vi "Spectrometer_R&S_2017.03.17.vi"(6 "ESR_stack_ref":refnum<vi>, 8 "current_run_ref":refnum<vi>, 9 "generator_enable":bool, 10 "sweep_parameters":T1={"Repetitions"=1, "Power dBm"=5.999999061226845, "Freq Start [Hz]"=2800000000.0, "Freq Stop [Hz]"=3000000000.0, "Step size [Hz]"=2500000.0, "Dwell Time [ms]"=0.09999999974525053} {"Dwell Time [ms]" format="%.3f"; "Step size [Hz]" format="%.2p"; "Freq Stop [Hz]" format="%.2p"; "Freq Start [Hz]" format="%.2p"; "Power dBm" format="%.2f"; "Repetitions" min=1 max=1000 step=1}, 11 "position_xyz":T2 {"Position Z" min=0.0 max=10.0 step=0.001 format="%.3f"; "Position Y" min=-10.0 max=10.0 step=0.1 format="%.3f"; "Position X" min=-10.0 max=10.0 step=0.1 format="%.3f"}) -> ()   [LabVIEW 2014]
uses:
  <vilib>/DAQmx/write.llb/DAQmx Write (Digital Bool 1Line 1Point).vi
  <vilib>/Analysis/baseanly.llb/Vector x A.vi
  GLOBAL_VAR.vi
  <vilib>/DAQmx/miscellaneous.llb/DAQmx Fill In Error Info.vi
  <vilib>/Analysis/Matrix/Numeric/Conversions/Array To Matrix - RA2.vi
  <vilib>/DAQmx/create/channels.llb/DAQmx Create Channel (CO-Pulse Generation-Ticks).vi
  <vilib>/DAQmx/create/channels.llb/DAQmx Create Channel (DO-Digital Output).vi
  <vilib>/DAQmx/create/channels.llb/DAQmx Create Channel (AO-Voltage-Basic).vi
  <vilib>/DAQmx/configure/trigger.llb/DAQmx Start Trigger (Digital Edge).vi
  <resource>/objmgr/daqmx.rc
  <vilib>/Analysis/NI_AALBase.lvlib
  <vilib>/Analysis/Matrix/NI_Matrix.lvlib
  <instrlib>/Rohde&Schwarz RF Signal Generator/Rohde&Schwarz RF Signal Generator.lvlib
  <vilib>/DAQmx/write.llb/DAQmx Write (Analog 1D DBL NChan 1Samp).vi
panel:
  out "File name":string
  in  "Save":bool
  in  "Stop":bool
  out "Run":i32=100
  out "Remain":i32
  out "Intensity Graph":ext[][](graph)
  out "Histogram":cluster{ext[], ext[]}[](graph)=[{[2700000000.0, 2702500000.0, 2705000000.0, 2707500000.0, 2710000000.0, 2712500000.0, 2715000000.0, 2717500000.0, 2720000000.0, 2722500000.0, 2725000000.0, 2727500000.0, 2730000000.0, 2732500000.0, 2735000000.0, 2737500000.0, 2740000000.0, 2742500000.0, 2745000000.0, 2747500000.0, 2750000000.0, 2752500000.0, 2755000000.0, 2757500000.0, 2760000000.0, 2762500000.0, 2765000000.0, 2767500000.0, 2770000000.0, 2772500000.0, 2775000000.0, 2777500000.0, 2780000000.0, 2782500000.0, 2785000000.0, 2787500000.0, 2790000000.0, 2792500000.0, 2795000000.0, 2797500000.0, 2800000000.0, 2802500000.0, 2805000000.0, 2807500000.0, 2810000000.0, 2812500000.0, 2815000000.0, 2817500000.0, 2820000000.0, 2822500000.0, 2825000000.0, 2827500000.0, 2830000000.0, 2832500000.0, 2835000000.0, 2837500000.0, 2840000000.0, 2842500000.0, 2845000000.0, 2847500000.0, 2850000000.0, 2852500000.0, 2855000000.0, 2857500000.0, 2860000000.0, 2862500000.0, 2865000000.0, 2867500000.0, 2870000000.0, 2872500000.0, 2875000000.0, 2877500000.0, 2880000000.0, 2882500000.0, 2885000000.0, 2887500000.0, 2890000000.0, 2892500000.0, 2895000000.0, 2897500000.0, 2900000000.0, 2902500000.0, 2905000000.0, 2907500000.0, 2910000000.0, 2912500000.0, 2915000000.0, 2917500000.0, 2920000000.0, 2922500000.0, 2925000000.0, 2927500000.0, 2930000000.0, 2932500000.0, 2935000000.0, 2937500000.0, 2940000000.0, 2942500000.0, 2945000000.0, 2947500000.0, 2950000000.0, 2952500000.0, 2955000000.0, 2957500000.0, 2960000000.0, 2962500000.0, 2965000000.0, 2967500000.0, 2970000000.0, 2972500000.0, 2975000000.0, 2977500000.0, 2980000000.0, 2982500000.0, 2985000000.0, 2987500000.0, 2990000000.0, 2992500000.0, 2995000000.0, 2997500000.0, 3000000000.0], [26841.121559672197128, 27464.174520667373477, 27576.32405364650522, 29408.099758972323686, 27638.629349746022854, 27576.32405364650522, 27638.629349746022854, 27651.09040896592638, 28398.753962160138, 28311.526547620813311, 28236.76019230139215, 27912.772652583900449, 27850.467356484382814, 27875.389474924189868, 28174.454896201874515, 28697.819383437822648, 28685.35832421791912, 28535.825613579076798, 28809.968916416954391, 29046.729041595121403, 28647.975146558208541, 28523.36455435917327, 28062.305363222742772, 28174.454896201874515, 28473.520317479559163, 27738.31782350525107, 28423.676080599945054, 29133.956456134446093, 28859.8131532965685, 27638.629349746022854, 29133.956456134446093, 27763.239941945058124, 27352.024987688241733, 27439.252402227566423, 28822.429975636857918, 27526.479816766891112, 28548.286672798980325, 27838.006297264479286, 28847.352094076664972, 28884.735271736375553, 29271.02810755338489, 28884.735271736375553, 27289.7196915887241, 28971.962686275700243, 28336.448666060620365, 28548.286672798980325, 27975.077948683418082, 27763.239941945058124, 29470.405055071841321, 28822.429975636857918, 28087.227481662549826, 28286.604429181006259, 27352.024987688241733, 27401.869224567855841, 28398.753962160138, 29308.411285213095471, 28485.98137669946269, 28585.669850458690906, 28710.280442657726175, 28236.76019230139215, 28311.526547620813311, 27576.32405364650522, 27302.180750808627625, 28299.065488400909786, 26878.504737331907709, 28809.968916416954391, 29420.560818192227213, 28859.8131532965685, 27750.778882725154597, 28535.825613579076798, 28398.753962160138, 28261.682310741199204, 28947.040567835893189, 28361.370784500427419, 28785.046797977147337, 28610.59196889849796, 27476.635579887277004, 28062.305363222742772, 28311.526547620813311, 28809.968916416954391, 28647.975146558208541, 28112.14960010235688, 28822.429975636857918, 27738.31782350525107, 28199.377014641681569, 28510.903495139269744, 27451.71346144746995, 28074.766422442646299, 27725.856764285347543, 28635.514087338305014, 28834.891034856761445, 27376.947106128048787, 29096.573278474735512, 28274.143369961102731, 29034.267982375217876, 28560.747732018883852, 27277.258632368820573, 28884.735271736375553, 28049.844304002839245, 27975.077948683418082, 26965.732151871232396, 28809.968916416954391, 28000.000067123225136, 27127.725921729978248, 28037.383244782935718, 28000.000067123225136, 27277.258632368820573, 27800.623119604768705, 28087.227481662549826, 27501.557698327084058, 26778.816263572679492, 26429.906605415380737, 27526.479816766891112, 26442.367664635284264, 26479.750842294994845, 27775.701001164961651, 27040.498507190653559, 26429.906605415380737, 27750.778882725154597, 27464.174520667373477, 27925.233711803803976]}, {[2700000000.0, 2702500000.0, 2705000000.0, 2707500000.0, 2710000000.0, 2712500000.0, 2715000000.0, 2717500000.0, 2720000000.0, 2722500000.0, 2725000000.0, 2727500000.0, 2730000000.0, 2732500000.0, 2735000000.0, 2737500000.0, 2740000000.0, 2742500000.0, 2745000000.0, 2747500000.0, 2750000000.0, 2752500000.0, 2755000000.0, 2757500000.0, 2760000000.0, 2762500000.0, 2765000000.0, 2767500000.0, 2770000000.0, 2772500000.0, 2775000000.0, 2777500000.0, 2780000000.0, 2782500000.0, 2785000000.0, 2787500000.0, 2790000000.0, 2792500000.0, 2795000000.0, 2797500000.0, 2800000000.0, 2802500000.0, 2805000000.0, 2807500000.0, 2810000000.0, 2812500000.0, 2815000000.0, 2817500000.0, 2820000000.0, 2822500000.0, 2825000000.0, 2827500000.0, 2830000000.0, 2832500000.0, 2835000000.0, 2837500000.0, 2840000000.0, 2842500000.0, 2845000000.0, 2847500000.0, 2850000000.0, 2852500000.0, 2855000000.0, 2857500000.0, 2860000000.0, 2862500000.0, 2865000000.0, 2867500000.0, 2870000000.0, 2872500000.0, 2875000000.0, 2877500000.0, 2880000000.0, 2882500000.0, 2885000000.0, 2887500000.0, 2890000000.0, 2892500000.0, 2895000000.0, 2897500000.0, 2900000000.0, 2902500000.0, 2905000000.0, 2907500000.0, 2910000000.0, 2912500000.0, 2915000000.0, 2917500000.0, 2920000000.0, 2922500000.0, 2925000000.0, 2927500000.0, 2930000000.0, 2932500000.0, 2935000000.0, 2937500000.0, 2940000000.0, 2942500000.0, 2945000000.0, 2947500000.0, 2950000000.0, 2952500000.0, 2955000000.0, 2957500000.0, 2960000000.0, 2962500000.0, 2965000000.0, 2967500000.0, 2970000000.0, 2972500000.0, 2975000000.0, 2977500000.0, 2980000000.0, 2982500000.0, 2985000000.0, 2987500000.0, 2990000000.0, 2992500000.0, 2995000000.0, 2997500000.0, 3000000000.0], [27662.305362263847, 27614.704116043806, 27558.75396014644, 27479.62623410005, 27635.264863756656, 27635.514084941045, 27523.73838373851, 27614.704116043802, 27583.17763621744, 27571.58885114293, 27593.520315369973, 27605.109100444486, 27505.545237277456, 27540.685424277577, 27573.831841802512, 27521.74461426332, 27747.788228512374, 27553.395704681883, 27408.099754177805, 27507.040564383846, 27553.769536458476, 27450.09352374888, 27547.16517507192, 27590.529661157172, 27485.98137430221, 27331.838071751987, 27460.06237112481, 27420.436202805507, 27402.99071989765, 27434.64181031619, 27576.697885423117, 27476.38635870286, 27470.654271461714, 27460.311592309215, 27451.962682631867, 27448.722807234688, 27469.781997316335, 27462.056140599987, 27364.23682572375, 27414.081062603364, 27456.573274543232, 27499.688539444087, 27488.598196738385, 27439.252402227583, 27451.215019078678, 27574.45489476352, 27513.894146954794, 27562.741499096825, 27559.377013107456, 27384.42374165998, 27576.074832462113, 27480.747729429848, 27504.423741947663, 27448.099754273695, 27508.90972326683, 27439.50162341197, 27397.383243248685, 27424.54835234809, 27331.21501879102, 27477.258632848276, 27459.68853934821, 27434.267978539607, 27381.05925567063, 27417.07171681613, 27347.912838145676, 27456.82249572762, 27392.398819560723, 27427.539006560855, 27402.86610930546, 27384.79757343659, 27482.86610949723, 27504.049910171063, 27508.037449121424, 27430.778881958024, 27495.202558124915, 27442.367667032533, 27426.16829004667, 27367.60131171313, 27402.616888121054, 27600.00006616432, 27539.68853953999, 27533.58262052224, 27462.305361784383, 27564.361436795392, 27572.087293511737, 27503.55146780227, 27476.137137518494, 27474.766421004293, 27580.560813781274, 27579.813150228085, 27592.024988263576, 27505.296016093063, 27570.84118758975, 27614.953337228195, 27611.215019462234, 27484.236826011424, 27503.925299578863, 27544.54835263575, 27602.616888600503, 27550.903492837893, 27593.769536554377, 27516.63557998317, 27611.962683015438, 27551.028103430108, 27655.701000877292, 27659.688539827646, 27578.5670443061, 27729.59508205134, 27610.093524132444, 27489.968913252564, 27615.202558412602, 27486.479816671, 27421.059255766515, 27418.56704392252, 27449.221249603488, 27600.996950901917, 27543.92529967475, 27425.17140530909, 27466.04367955036, 27523.987604922913, 27501.183866550484]}]
  in  "start":bool
  in  "stop":bool
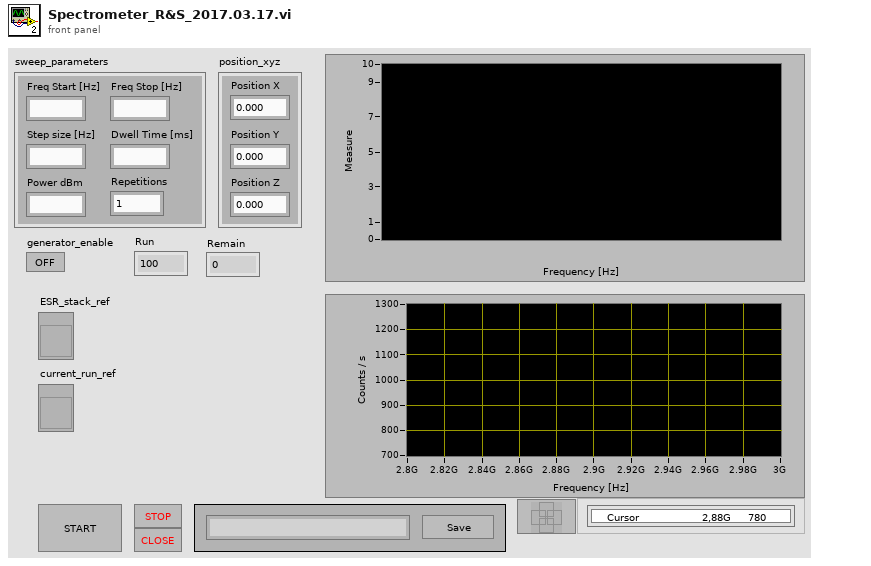
[diagram p1: front panel]
types:
  T1 = cluster{"Repetitions":i32, "Power dBm":ext, "Freq Start [Hz]":ext, "Freq Stop [Hz]":ext, "Step size [Hz]":ext, "Dwell Time [ms]":ext}
  T2 = cluster{"Position X":dbl, "Position Y":dbl, "Position Z":dbl}
  T3 = enum16{"stand-by", "init", "config", "acquisition", "processing", "close", "Set Variables"}
  T4 = typedef "NI_Matrix.lvlib/RealMatrix.ctl" = dbl[][]
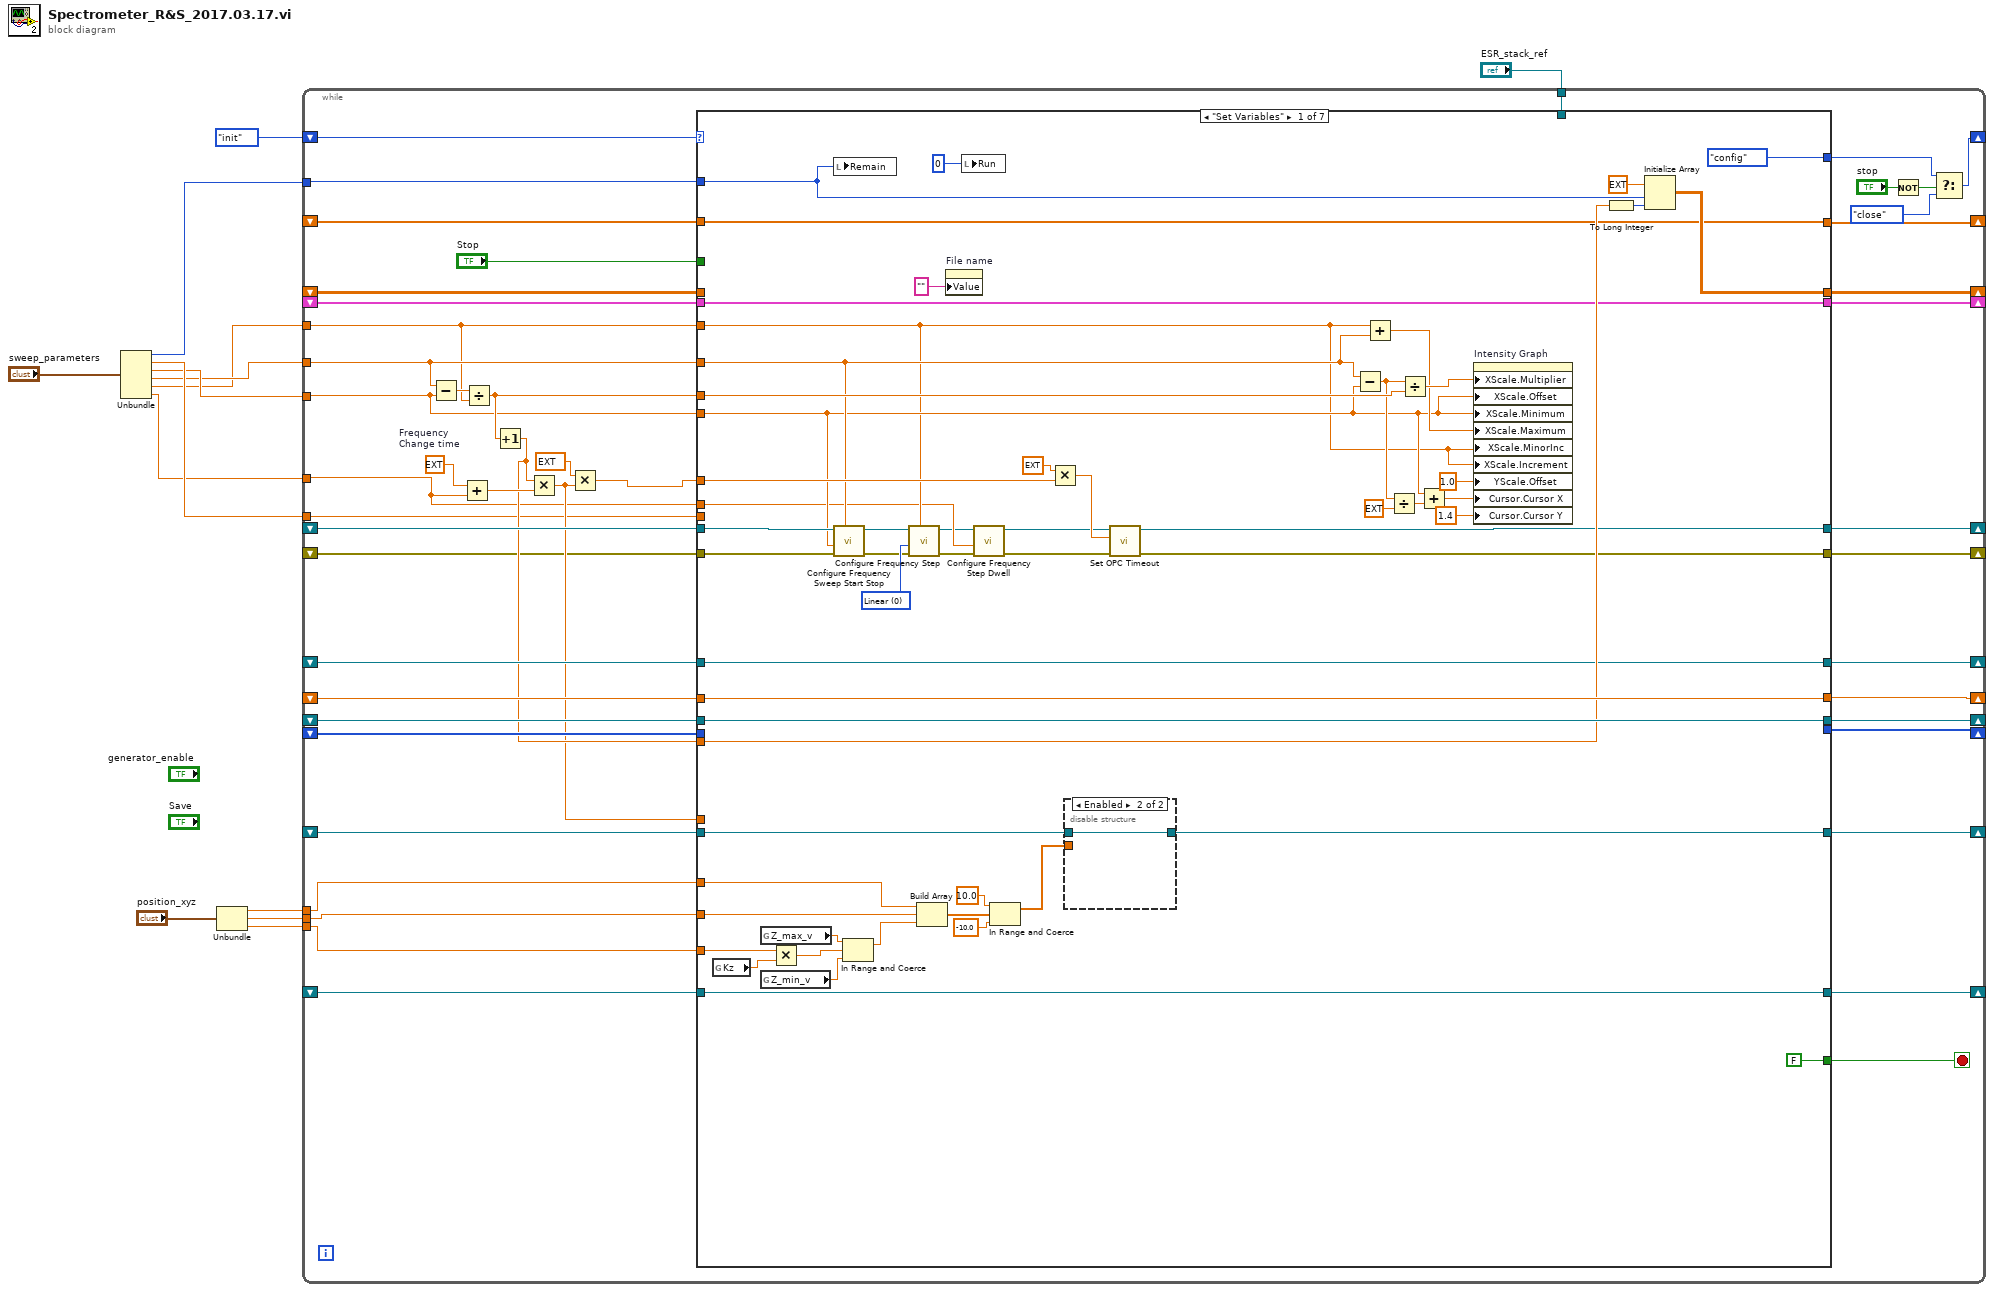
[diagram p0: block diagram]
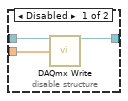
[diagram p2: hidden frame]
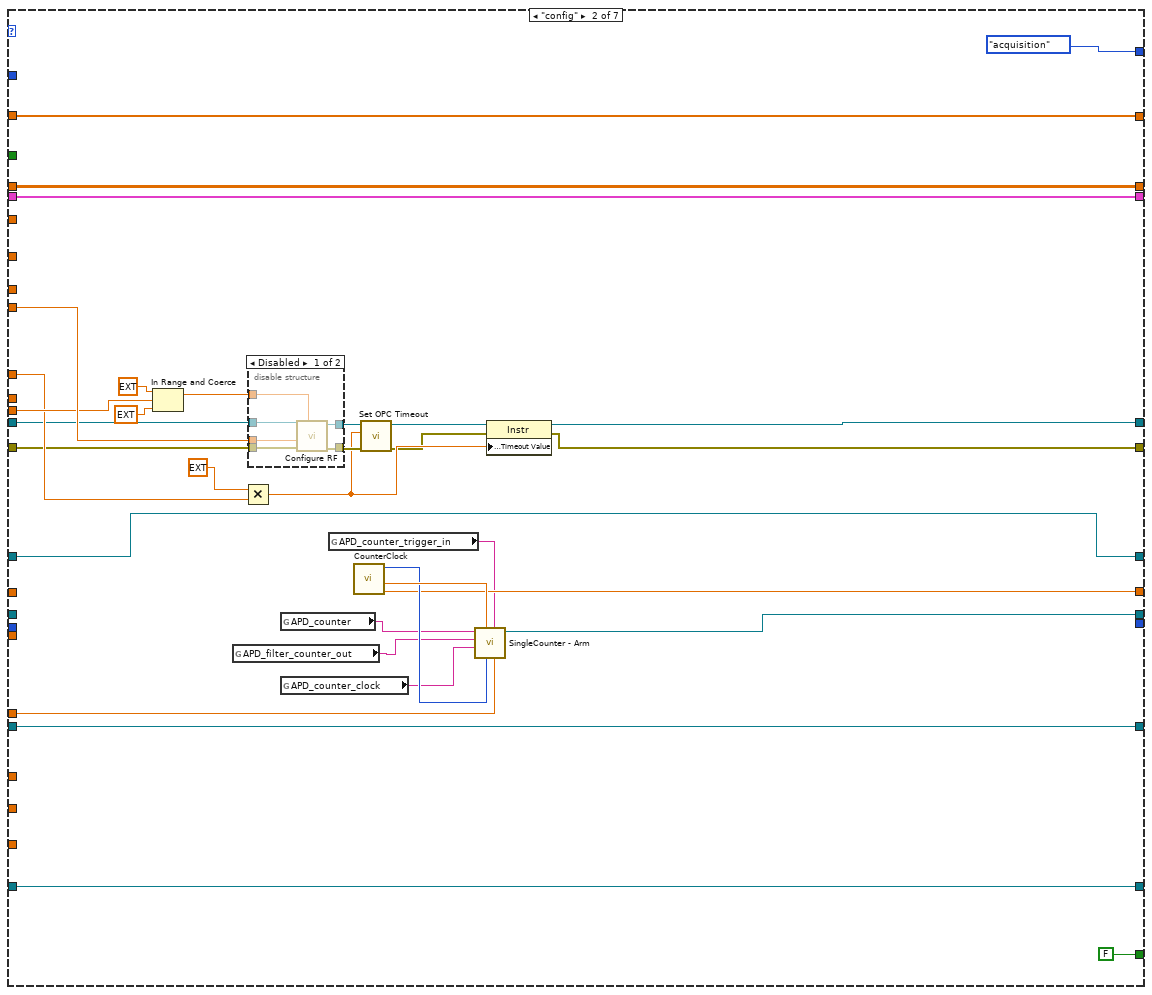
[diagram p3: hidden frame]
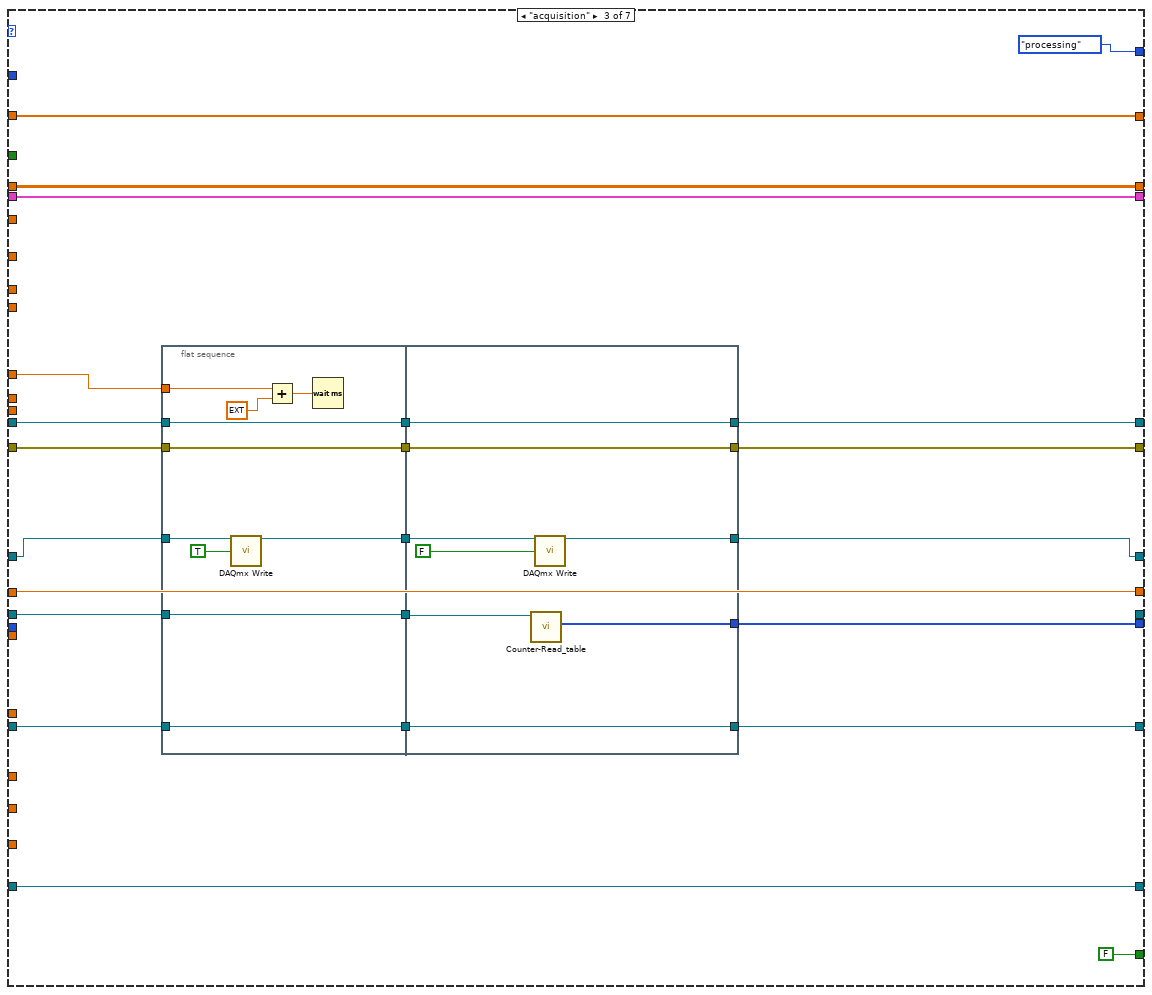
[diagram p5: hidden frame]
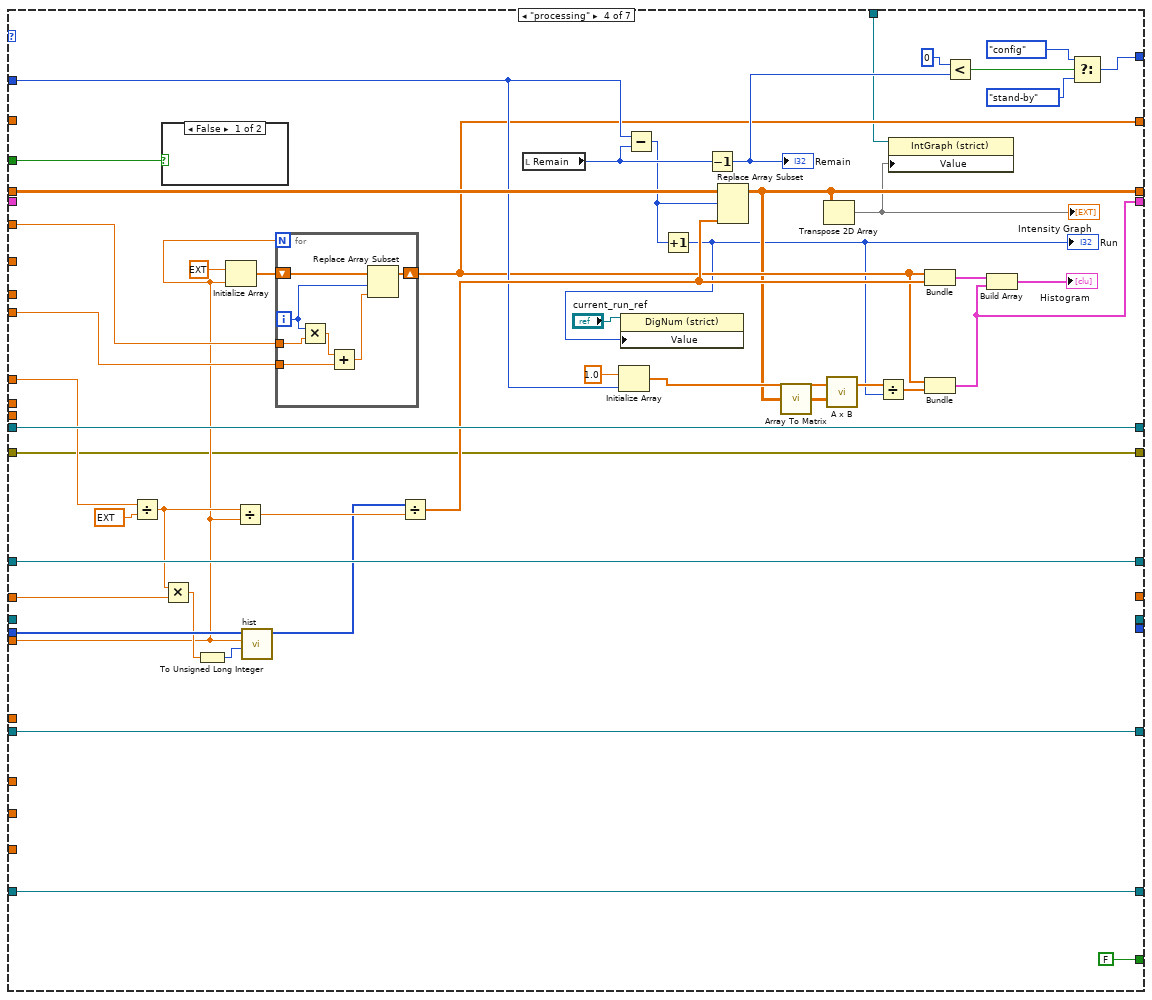
[diagram p6: hidden frame]
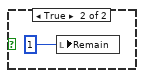
[diagram p7: hidden frame]
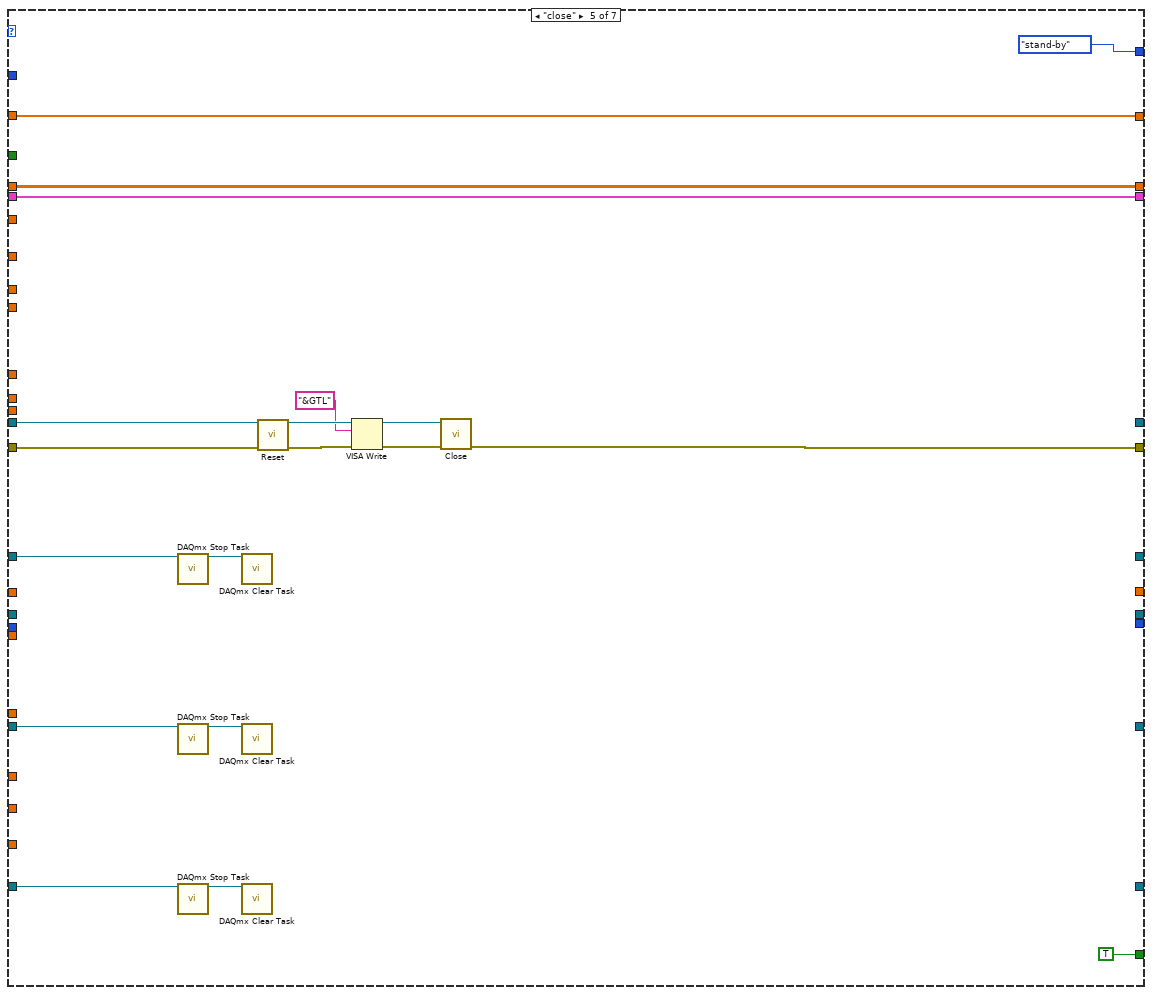
[diagram p8: hidden frame]
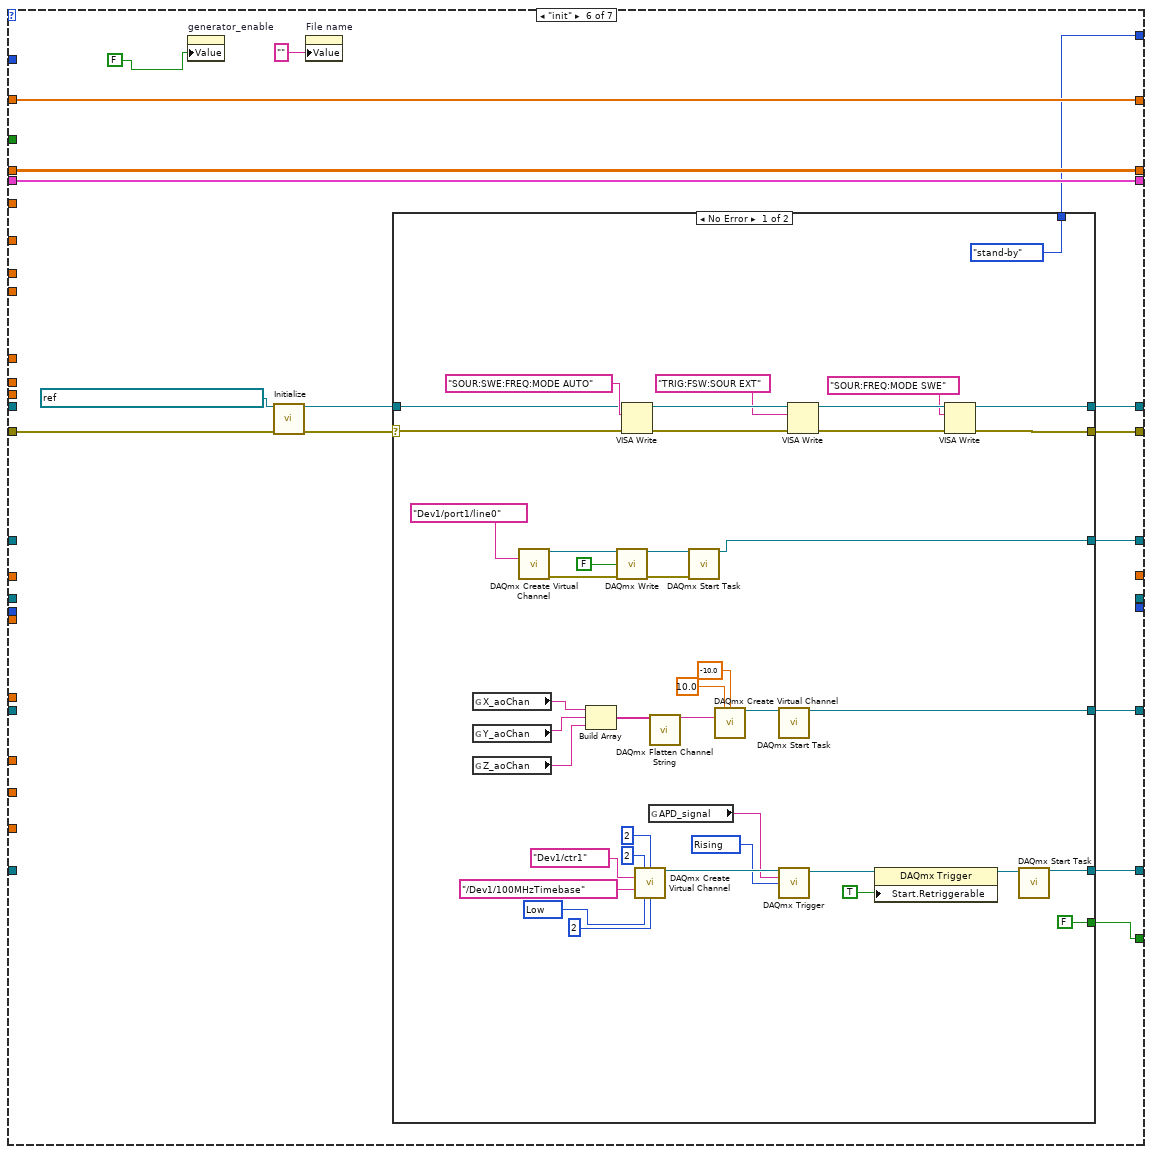
[diagram p9: hidden frame]
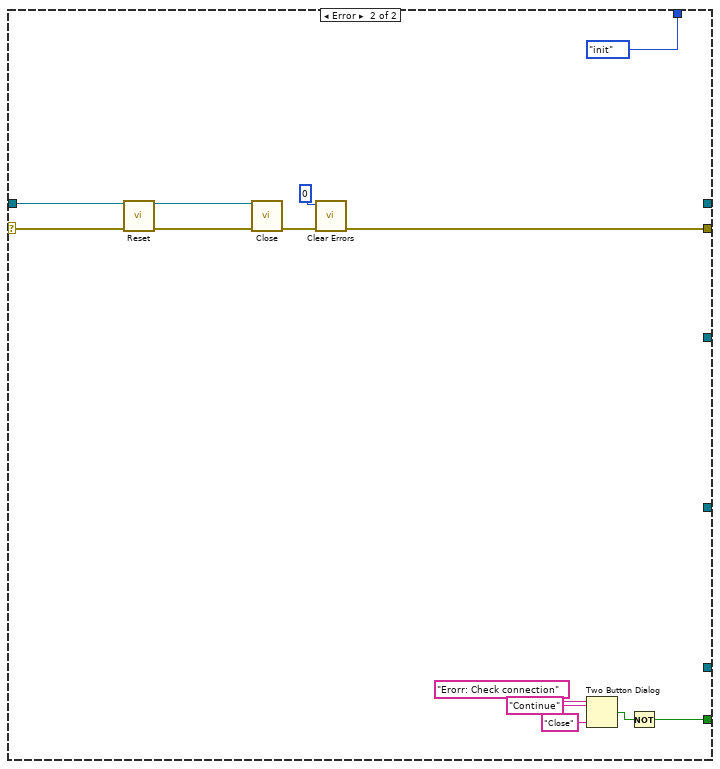
[diagram p10: hidden frame]
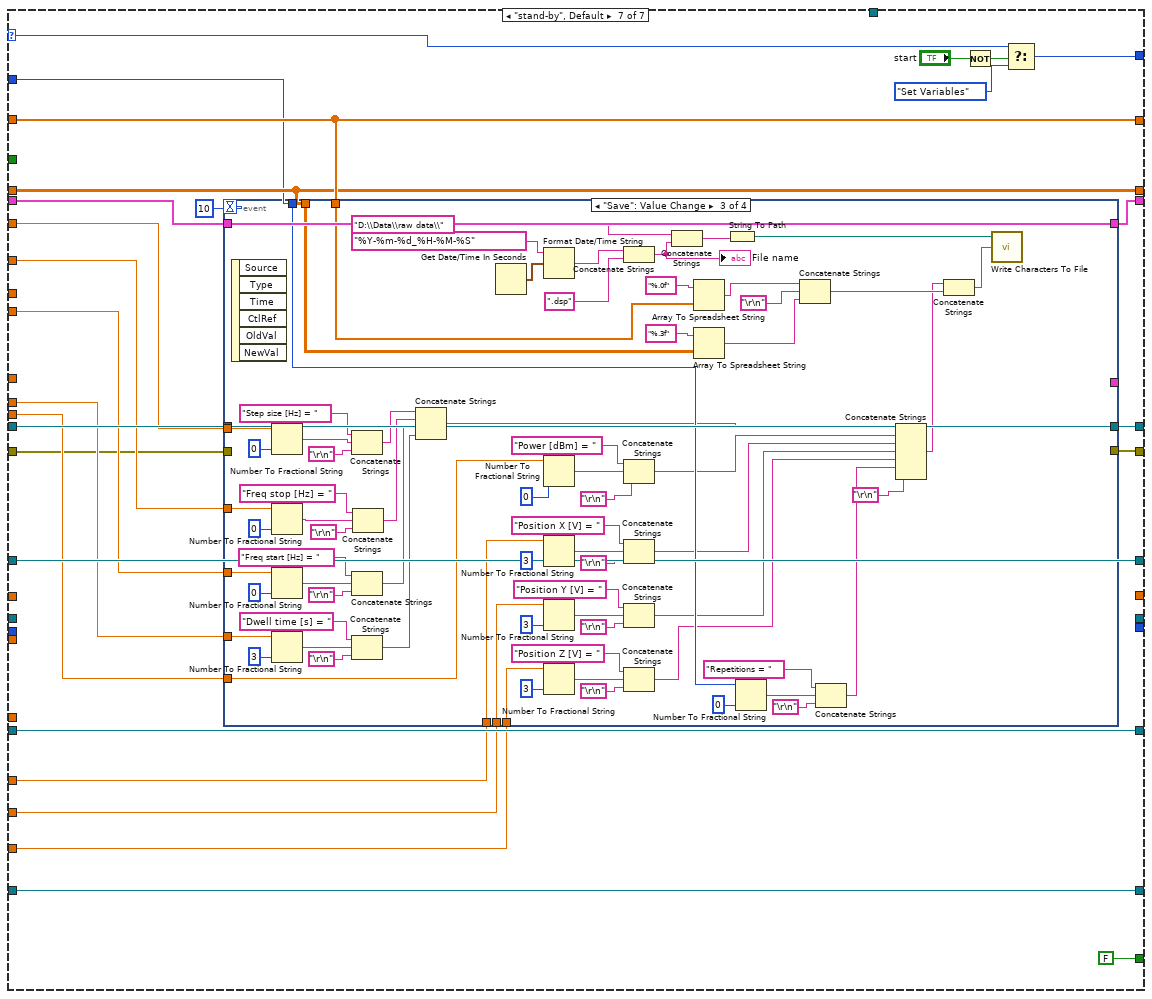
[diagram p11: hidden frame]
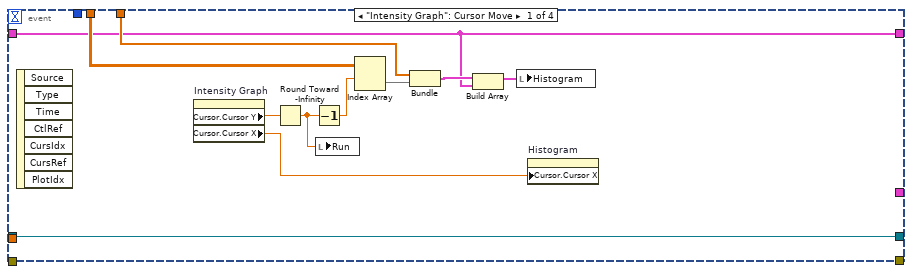
[diagram p12: hidden frame]
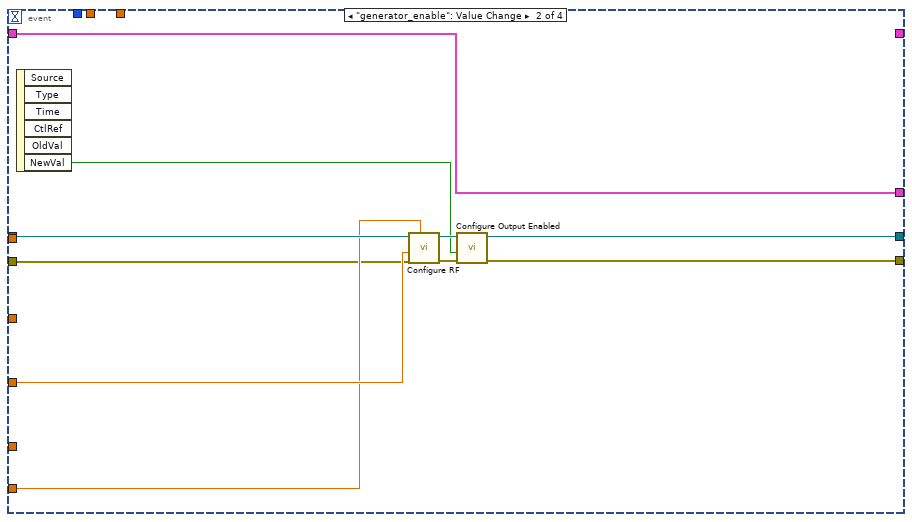
[diagram p13: hidden frame]
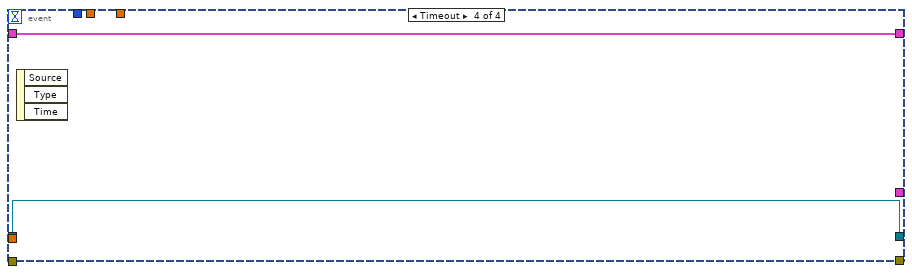
[diagram p14: hidden frame]
diagram:
  n1 = Unbundle("sweep_parameters") -> ("Repetitions"=w7:i32, "Power dBm"=w6:ext, "Freq Start [Hz]"=w5:ext, "Freq Stop [Hz]"=w4:ext, "Step size [Hz]"=w3:ext, "Dwell Time [ms]"=w2:ext)
  n2 = Unbundle("position_xyz") -> ("Position X"=w11:dbl, "Position Y"=w10:dbl, "Position Z"=w9:dbl)
  n3 = while {
    shift-right: [w47] -> _
    shift-left: T3."init" -> [w61]
    shift-right: [w57] -> _
    shift-left: _ -> [w56]
    shift-right: [w27] -> _
    shift-left: _ -> [w55]
    shift-right: [w54] -> _
    shift-left: _ -> [w53]
    shift-right: [w52] -> _
    shift-left: _ -> [w51]
    shift-right: [w45] -> _
    shift-left: _ -> [w44]
    shift-right: [w29] -> _
    shift-left: _ -> [w40]
    shift-right: [w37] -> _
    shift-left: _ -> [w39]
    shift-right: [w36] -> _
    shift-left: _ -> [w35]
    shift-right: [w33] -> _
    shift-left: _ -> [w32]
    shift-right: [w31] -> _
    shift-left: _ -> [w30]
    shift-right: [w26] -> _
    shift-left: _ -> [w25]
    tunnel: w11 -> [w23]
    tunnel: w10 -> [w22]
    tunnel: w9 -> [w21]
    tunnel: w7 -> [w20]
    tunnel: w6 -> [w19]
    tunnel: w5 -> [w18]
    tunnel: w4 -> [w17]
    tunnel: w3 -> [w16]
    tunnel: w2 -> [w15]
    tunnel: "ESR_stack_ref" -> [w14]
    stop <- w46 stop-if-true
    w24 = ext 0.0  # Frequency Change time
    n4 = Subtract(x=w17, y=w18) -> (x-y=w60:ext)
    n5 = Add(x=w24, y=w15) -> (x+y=w59:ext)
    n6 = Divide(x=w60, y=w16) -> (x/y=w41:ext)
    n7 = Increment(x=w41) -> (x+1=w42:ext)
    n8 = Multiply(x=w42, y=w59) -> (x*y=w34:ext)
    n9 = Multiply(x=ext 1000.0 ("y"), y=w34) -> (x*y=w58:ext)
    n10 = case shown="\"Set Variables\"" w61 {
      selector: w61 -> [_ _ _ _ _ _ w374]
      tunnel: [T3."config" T3."acquisition" T3."processing" w234 T3."stand-by" w283 w373] -> w48
      tunnel: [w68 w129 w184 w243 _ w285 w359] -> w57
      tunnel: [w84 w154 w169 w242 _ w284 w371] -> w27
      tunnel: w56 -> [w87 w134 w185 w243 w272 _ w360]
      tunnel: w55 -> [w84 w154 w170 w242 w276 _ w371]
      tunnel: w16 -> [w77 _ _ w241 _ _ w358]
      tunnel: w17 -> [w81 _ _ _ _ _ w357]
      tunnel: w18 -> [w80 w140 _ w227 _ _ w356]
      tunnel: w58 -> [w85 w136 w168 w237 _ _ _]
      tunnel: w15 -> [w76 _ _ _ _ _ w355]
      tunnel: [w113 w150 _ _ _ _ _] -> w54
      tunnel: w53 -> [w113 _ w183 _ _ _ _]
      tunnel: [_ _ w182 _ _ _ _] -> w52
      tunnel: w51 -> [_ _ _ w248 _ _ _]
      tunnel: [FALSE FALSE FALSE FALSE TRUE w280 FALSE] -> w46
      tunnel: [w112 w149 w180 _ _ _ _] -> w45
      tunnel: w44 -> [w112 _ w180 w246 _ _ _]
      tunnel: w42 -> [w109 _ _ w222 _ _ _]
      tunnel: w41 -> [w108 _ _ _ _ _ _]
      tunnel: w19 -> [_ w137 _ _ _ _ w354]
      tunnel: w23 -> [w90 _ _ _ _ _ w353]
      tunnel: w40 -> [w95 w142 w179 w238 w273 _ w369]
      tunnel: w22 -> [w89 _ _ _ _ _ w352]
      tunnel: w21 -> [w66 _ _ _ _ _ w351]
      tunnel: w20 -> [w99 _ _ w219 _ _ w350]
      tunnel: w39 -> [_ w148 w177 w231 w271 w292 w364]
      tunnel: [w111 w148 w177 w211 w271 w292 w364] -> w37
      tunnel: [w100 w146 w175 w217 w269 w291 w366] -> w36
      tunnel: w35 -> [w100 w146 w175 _ w269 w291 w366]
      tunnel: w34 -> [_ w145 _ _ _ _ _]
      tunnel: [w97 w144 w174 w224 _ w281 w363] -> w33
      tunnel: w32 -> [w97 w144 w174 w224 w267 _ w363]
      tunnel: [w96 w143 w173 w209 w266 w290 w361] -> w31
      tunnel: w30 -> [w96 w143 w173 _ w266 w290 w362]
      tunnel: [w94 w142 w178 w238 _ w282 w369] -> w29
      tunnel: "Stop" -> [_ _ _ w212 _ _ _]
      tunnel: [w67 w126 w171 w210 w263 w279 w348] -> w26
      tunnel: w25 -> [w78 w132 w172 w210 w264 w278 w349]
      tunnel: w14 -> [_ _ _ w207 _ _ _]
      frame "Set Variables" {
        w75 = 0 items=["Linear", "Logarithmic"] ("Scaling (Linear)")
        n11 = global read "GLOBAL_VAR.vi" "Kz"() -> (w64:dbl)
        n12 = global read "GLOBAL_VAR.vi" "Z_max_v"() -> (w63:dbl)
        n13 = global read "GLOBAL_VAR.vi" "Z_min_v"() -> (w62:dbl)
        n14 = Multiply(x=w66, y=w64) -> (x*y=w65:dbl)
        n15 = local write "Remain"(w99) -> ()
        n16 = call <instrlib>:"Configure Frequency Sweep Start Stop.vi"("Stop (500.0e6)"=w81, "error in (no error)"=w78, "Start (100.0e6)"=w80, "VISA resource name"=w87) -> ("error out"=w73:errorcluster, "VISA resource name out"=w74:refnum<visa-resource-name>)  [unwired: 6 in]
        n17 = In Range and Coerce(upper limit=w63, x=w65, lower limit=w62) -> (coerced(x)=w92:dbl)  [unwired: 1 out]
        n18 = call <instrlib>:"Configure Frequency Step.vi"("Step Size (100.0e3)"=w77, "error in (no error)"=w73, "Scaling (Linear)"=w75, "VISA resource name"=w74) -> ("error out"=w71:errorcluster, "VISA resource name out"=w72:refnum<visa-resource-name>)  [unwired: 6 in]
        n19 = Build Array(w90, w89, w92) -> (w91:dbl[])
        n20 = property on="File name" class="Str"("Value"="" ("File name")) -> ()  [unwired: 2 in, 2 out]
        n21 = local write "Run"(0 ("Run")) -> ()
        n22 = call <instrlib>:"Configure Frequency Step Dwell.vi"("error in (no error)"=w71, "Dwell (10.0e-3)"=w76, "VISA resource name"=w72) -> ("error out"=w69:errorcluster, "VISA resource name out"=w70:refnum<visa-resource-name>)  [unwired: 7 in]
        n23 = In Range and Coerce(upper limit=10.0, x=w91, lower limit=-10.0) -> (coerced(x)=w88:dbl[])  [unwired: 1 out]
        n24 = Multiply(x=ext 1.100000023841858, y=w85) -> (x*y=w79:ext)
        n25 = disable-structure shown="Enabled" {
          disable-tunnel: w95 -> [w120 w121]
          disable-tunnel: [w119 w121] -> w94
          disable-tunnel: w88 -> [w118 _]
          frame Disabled {
            n26 = call-poly <vilib>:"DAQmx Write.vi"("task/channels in"=w120, "data"=w118) -> ("task out"=w119:refnum<k21>)  [unwired: 11 in, 2 out]
          }
          frame Enabled {
          }
        }
        n27 = call <instrlib>:"Set OPC Timeout.vi"("error in (no error)"=w69, "OPC Timeout (0)"=w79, "VISA resource name"=w70) -> ("error out"=w67:errorcluster, "VISA resource name out"=w68:refnum<visa-resource-name>)  [unwired: 7 in]
        n28 = Subtract(x=w81, y=w80) -> (x-y=w105:ext)
        n29 = Add(x=w77, y=w81) -> (x+y=w107:ext)
        n30 = Divide(x=w105, y=ext 2.0) -> (x/y=w101:ext)
        n31 = Divide(x=w105, y=w108) -> (x/y=w110:ext)
        n32 = Add(x=w80, y=w101) -> (x+y=w102:ext)
        n33 = property on="Intensity Graph" class="IntGraph (strict)"("XScale.Multiplier"=w110, "XScale.Offset"=w80, "XScale.Minimum"=w80, "XScale.Maximum"=w107, "XScale.MinorInc"=w77, "XScale.Increment"=w77, "YScale.Offset"=1.0 ("Y Scale.Offset and Multiplier:Offset"), "Cursor.Cursor X"=w102, "Cursor.Cursor Y"=1.4 ("Cursor.Cursor Position:Cursor Y")) -> ()  [unwired: 2 in, 2 out]
        n34 = To Long Integer(number=w109) -> (32bit integer=w115:i32)
        n35 = Initialize Array(ext 0.0 ("element"), w99, w115) -> (w111:ext[][])
      }
      frame "config" {
        n36 = In Range and Coerce(upper limit=ext 27.0, x=w137, lower limit=ext -36.0) -> (coerced(x)=w141:ext)  [unwired: 1 out]
        n37 = global read "GLOBAL_VAR.vi" "APD_filter_counter_out"() -> (w122:tag)
        n38 = Multiply(x=ext 5.0 ("lower limit"), y=w136) -> (x*y=w128:ext)
        n39 = disable-structure shown="Disabled" {
          disable-tunnel: w141 -> [w160 _]
          disable-tunnel: w140 -> [w159 _]
          disable-tunnel: w134 -> [w158 w162]
          disable-tunnel: [w157 w162] -> w133
          disable-tunnel: w132 -> [w156 w161]
          disable-tunnel: [w155 w161] -> w131
          frame Disabled {
            n40 = call <instrlib>:"Configure RF.vi"("Power Level (-30.0)"=w160, "error in (no error)"=w156, "Frequency (1.0e9)"=w159, "VISA resource name"=w158) -> ("error out"=w155:errorcluster, "VISA resource name out"=w157:refnum<visa-resource-name>)  [unwired: 6 in]
          }
          frame Enabled {
          }
        }
        n41 = global read "GLOBAL_VAR.vi" "APD_counter"() -> (w124:tag)
        n42 = global read "GLOBAL_VAR.vi" "APD_counter_clock"() -> (w123:tag)
        n43 = global read "GLOBAL_VAR.vi" "APD_counter_trigger_in"() -> (w125:tag)
        n44 = call "CounterClock.vi"() -> ("Counter clock rate divided by prescaler"=w149:dbl, "Counter clock rate"=w152:dbl, "CI.Prescaler"=w151:u32)  [unwired: 8 in, 1 out]
        n45 = call <instrlib>:"Set OPC Timeout.vi"("error in (no error)"=w131, "OPC Timeout (0)"=w128, "VISA resource name"=w133) -> ("error out"=w127:errorcluster, "VISA resource name out"=w130:refnum<visa-resource-name>)  [unwired: 7 in]
        n46 = call "SingleCounter - Arm.vi"("Duration"=w145, "Trigger Source"=w125, "CI.Prescaler"=w151, "Sampling Rate"=w152, "Clock Source"=w123, "External Timing Source"=w122, "counter"=w124) -> ("task out"=w150:refnum<k21>)  [unwired: 3 in, 1 out]
        n47 = property class="Instr"(reference=w130, error in=w127, "General Settings:Timeout Value"=w128) -> (reference out=w129:refnum<visa-resource-name>, error out=w126:errorcluster)
      }
      frame "acquisition" {
        n48 = flat-sequence {
          tunnel: w185 -> [w190]
          tunnel: [w194] -> w167
          tunnel: [w193] -> w166
          tunnel: w183 -> [w193]
          tunnel: [w192] -> w165
          tunnel: w179 -> [w192]
          tunnel: w172 -> [w189]
          tunnel: w170 -> [w191]
          tunnel: w168 -> [w187]
          tunnel: [w190] -> w164
          tunnel: [w189] -> w163
          tunnel: [w198] -> w169
          tunnel: [w197] -> w184
          tunnel: w167 -> [w202]
          tunnel: w166 -> [w200]
          tunnel: [w201] -> w182
          tunnel: [w199] -> w178
          tunnel: w165 -> [w199]
          tunnel: [w196] -> w171
          tunnel: w164 -> [w197]
          tunnel: w163 -> [w196]
          frame #0 {
            n49 = call-poly <vilib>:"DAQmx Write.vi"("task/channels in"=w191, "data"=TRUE) -> ("task out"=w194:refnum<k21>)  [unwired: 11 in, 2 out]
            n50 = Add(x=w187, y=ext 1.1) -> (x+y=w188:ext)
            n51 = Wait (ms)(milliseconds to wait=w188) -> ()  [unwired: 1 out]
          }
          frame #1 {
            n52 = call "Counter-Read_table.vi"("task in"=w200) -> ("time tags"=w201:u32[])  [unwired: 9 in, 1 out]
            n53 = call-poly <vilib>:"DAQmx Write.vi"("task/channels in"=w202, "data"=FALSE) -> ("task out"=w198:refnum<k21>)  [unwired: 11 in, 2 out]
          }
        }
      }
      frame "processing" {
        n54 = Divide(x=w237, y=ext 1000.0) -> (x/y=w236:ext)
        n55 = case shown="False" w212 {
          frame False {
          }
          frame True {
            n56 = local write "Remain"(1) -> ()
          }
        }
        n57 = Multiply(x=w236, y=w246) -> (x*y=w244:ext)
        n58 = To Unsigned Long Integer(number=w244) -> (unsigned 32bit integer=w245:u32)
        n59 = Initialize Array(ext 0.0 ("element"), w222) -> (w239:ext[])
        n60 = Divide(x=w236, y=w222) -> (x/y=w235:ext)
        n61 = call "hist.vi"("#clock cycles"=w245, "#bins"=w222, "counter timetag list"=w248) -> ("histogram"=w208:i32[])  [unwired: 7 in]
        n62 = for {
          N: w222 -> [_]
          tunnel: w241 -> [w253]
          shift-right: [w257] -> w217
          shift-left: w239 -> [w256]
          tunnel: w227 -> [w255]
          i -> [w254]
          n63 = Multiply(x=w254, y=w253) -> (x*y=w252:ext)
          n64 = Add(x=w252, y=w255) -> (x+y=w251:ext)
          n65 = Replace Array Subset(array=w256, new element=w251, index=w254) -> (w257:ext[])
        }
        n66 = Divide(x=w208, y=w235) -> (x/y=w223:ext[])
        n67 = local read "Remain"() -> (w226:i32)
        n68 = Initialize Array(1.0 ("element"), w219) -> (w218:dbl[])
        n69 = Subtract(x=w219, y=w226) -> (x-y=w225:i32)
        n70 = Increment(x=w225) -> (x+1=w204:i32)
        "Run" <- w204
        n71 = property class="DigNum (strict)"(reference="current_run_ref", "Value"=w204) -> ()  [unwired: 1 in, 2 out]
        n72 = Decrement(x=w226) -> (x-1=w228:i32)
        "Remain" <- w228
        n73 = Replace Array Subset(array=w231, new element=w223, index (row)=w225) -> (w211:ext[][])  [unwired: 1 in]
        n74 = call-poly <vilib>:"Array To Matrix.vi"("Real 2D Array"=w211) -> ("Real Matrix"=w221:T4)
        n75 = Transpose 2D Array(2D array=w211) -> (transposed array=w206:ext[][])
        "Intensity Graph" <- w206
        n76 = call-poly <vilib>:"A x B.vi"("Matrix A"=w221, "Vector V'"=w218) -> ("V' x A"=w215:dbl[])  [unwired: 1 out]
        n77 = Divide(x=w215, y=w204) -> (x/y=w216:dbl[])
        n78 = property class="IntGraph (strict)"(reference=w207, "Value"=w206) -> ()  [unwired: 1 in, 2 out]
        n79 = Bundle(w217, w223) -> (w214:cluster{ext[], ext[]})  [unwired: 1 in]
        n80 = Bundle(w217, w216) -> (w209:cluster{ext[], dbl[]})  [unwired: 1 in]
        n81 = Less?(x=0, y=w228) -> (x < y?=w232:bool)
        n82 = Build Array(w214, w209) -> (→"Histogram":cluster{ext[], ext[]}[])
        n83 = Select(t=T3."config", s=w232, f=T3."stand-by") -> (s? t:f=w234:T3)
      }
      frame "close" {
        n84 = call <vilib>:"DAQmx Stop Task.vi"("task/channels in"=w276) -> ("task out"=w275:refnum<k21>)  [unwired: 13 in, 1 out]
        n85 = call <vilib>:"DAQmx Stop Task.vi"("task/channels in"=w273) -> ("task out"=w265:refnum<k21>)  [unwired: 13 in, 1 out]
        n86 = call <vilib>:"DAQmx Stop Task.vi"("task/channels in"=w267) -> ("task out"=w268:refnum<k21>)  [unwired: 13 in, 1 out]
        n87 = call <vilib>:"DAQmx Clear Task.vi"("task in"=w275) -> ()  [unwired: 14 in, 1 out]
        n88 = call <vilib>:"DAQmx Clear Task.vi"("task in"=w265) -> ()  [unwired: 14 in, 1 out]
        n89 = call <vilib>:"DAQmx Clear Task.vi"("task in"=w268) -> ()  [unwired: 14 in, 1 out]
        n90 = call <instrlib>:"Reset.vi"("VISA resource name"=w272, "error in (no error)"=w264) -> ("VISA resource name out"=w262:refnum<visa-resource-name>, "error out"=w260:errorcluster)  [unwired: 12 in]
        n91 = VISA Write(VISA resource name=w262, write buffer="&GTL", error in (no error)=w260) -> (VISA resource name out=w261:refnum<visa-resource-name>, error out=w259:errorcluster)  [unwired: 1 out]
        n92 = call <instrlib>:"Close.vi"("error in (no error)"=w259, "VISA resource name"=w261) -> ("error out"=w263:errorcluster)  [unwired: 9 in]
      }
      frame "init" {
        n93 = property on="generator_enable" class="Bool (strict)"("Value"=FALSE ("Generator  output")) -> ()  [unwired: 2 in, 2 out]
        n94 = call <instrlib>:"Initialize.vi"("VISA resource name"=refnum<visa-resource-name> "USB0::0x0AAD::0x005F::262159::INSTR", "error in (no error)"=w278) -> ("VISA resource name out"=w286:refnum<visa-resource-name>, "error out"=w287:errorcluster)  [unwired: 12 in]
        n95 = property on="File name" class="Str"("Value"="" ("File name")) -> ()  [unwired: 2 in, 2 out]
        n96 = case shown="No Error" w287 {
          selector: w287 -> [w307 w346]
          tunnel: [w305 _] -> w285
          tunnel: w286 -> [w304 w347]
          tunnel: [w297 _] -> w284
          tunnel: [T3."stand-by" T3."init"] -> w283
          tunnel: [w328 _] -> w282
          tunnel: [w316 _] -> w281
          tunnel: [FALSE w338] -> w280
          tunnel: [w306 w335] -> w279
          frame No Error {
            w322 = 10280 items=["Rising"=10280, "Falling"=10171] ("edge")
            w318 = 10214 items=["High"=10192, "Low"=10214] ("idle state")
            n97 = global read "GLOBAL_VAR.vi" "X_aoChan"() -> (w296:tag)
            n98 = global read "GLOBAL_VAR.vi" "Y_aoChan"() -> (w294:tag)
            n99 = global read "GLOBAL_VAR.vi" "Z_aoChan"() -> (w295:tag)
            n100 = call-poly <vilib>:"DAQmx Create Virtual Channel.vi"("lines"=tag "Dev1/port1/line0") -> ("task out"=w298:refnum<k21>, "error out"=w301:errorcluster)  [unwired: 13 in]
            n101 = Build Array(w296, w294, w295) -> (w332:tag[])
            n102 = call-poly <vilib>:"DAQmx Write.vi"("task/channels in"=w298, "data"=FALSE, "error in"=w301) -> ("task out"=w300:refnum<k21>, "error out"=w302:errorcluster)  [unwired: 10 in, 1 out]
            n103 = VISA Write(VISA resource name=w304, write buffer="SOUR:SWE:FREQ:MODE AUTO", error in (no error)=w307) -> (VISA resource name out=w314:refnum<visa-resource-name>, error out=w311:errorcluster)  [unwired: 1 out]
            n104 = call-poly <vilib>:"DAQmx Create Virtual Channel.vi"("high ticks"=u32 2, "low ticks"=u32 2, "counter"=tag "Dev1/ctr1", "source of ticks"=tag "/Dev1/100MHzTimebase", "idle state"=w318, "initial delay"=u32 2) -> ("task out"=w327:refnum<k21>)  [unwired: 8 in, 1 out]
            n105 = global read "GLOBAL_VAR.vi" "APD_signal"() -> (w293:tag)
            n106 = call <vilib>:"DAQmx Flatten Channel String.vi"("names in"=w332) -> ("names out"=w333:string)  [unwired: 13 in, 1 out]
            n107 = call <vilib>:"DAQmx Start Task.vi"("task/channels in"=w300, "error in"=w302) -> ("task out"=w297:refnum<k21>)  [unwired: 12 in, 1 out]
            n108 = call-poly <vilib>:"DAQmx Create Virtual Channel.vi"("maximum value"=10.0, "minimum value"=-10.0, "physical channels"=w333) -> ("task out"=w331:refnum<k21>)  [unwired: 11 in, 1 out]
            n109 = call <vilib>:"DAQmx Start Task.vi"("task/channels in"=w331) -> ("task out"=w328:refnum<k21>)  [unwired: 13 in, 1 out]
            n110 = call-poly <vilib>:"DAQmx Trigger.vi"("task/channels in"=w327, "source"=w293, "edge"=w322) -> ("task out"=w323:refnum<k21>)  [unwired: 11 in, 1 out]
            n111 = VISA Write(VISA resource name=w314, write buffer="TRIG:FSW:SOUR EXT" ("write buffer 2"), error in (no error)=w311) -> (VISA resource name out=w313:refnum<visa-resource-name>, error out=w312:errorcluster)  [unwired: 1 out]
            n112 = property class="DAQmx Trigger"(reference=w323, "Start.Retriggerable"=TRUE) -> (reference out=w325:refnum<k21>)  [unwired: 1 in, 1 out]
            n113 = VISA Write(VISA resource name=w313, write buffer="SOUR:FREQ:MODE SWE" ("write buffer 3"), error in (no error)=w312) -> (VISA resource name out=w305:refnum<visa-resource-name>, error out=w306:errorcluster)  [unwired: 1 out]
            n114 = call <vilib>:"DAQmx Start Task.vi"("task/channels in"=w325) -> ("task out"=w316:refnum<k21>)  [unwired: 13 in, 1 out]
          }
          frame Error {
            n115 = call <instrlib>:"Reset.vi"("VISA resource name"=w347, "error in (no error)"=w346) -> ("VISA resource name out"=w337:refnum<visa-resource-name>, "error out"=w336:errorcluster)  [unwired: 12 in]
            n116 = call <instrlib>:"Close.vi"("error in (no error)"=w336, "VISA resource name"=w337) -> ("error out"=w342:errorcluster)  [unwired: 9 in]
            n117 = call <vilib>:"Clear Errors.vi"("error in (no error)"=w342, "specific error code to clear (0: all)"=0) -> ("error out"=w335:errorcluster)  [unwired: 4 in, 1 out]
            n118 = Two Button Dialog(message="Erorr: Check connection", 1:"Close" ("F button name (\"Cancel\")"), 2:"Continue" ("T button name (\"OK\")")) -> (T button?=w339:bool)
            n119 = Not(x=w339) -> (.not. x?=w338:bool)
          }
        }
      }
      frame "stand-by", Default {
        n120 = event shown="[2] \"Save\": Value Change" {
          selector: _ -> [_ _ _ _]
          dyn-events: _ -> [_ _ _ _]
          timeout: 10 -> [_ _ _ _]
          tunnel: w366 -> [w385 _ w461 _]
          tunnel: w364 -> [w381 _ w464 _]
          tunnel: w362 -> [w375 w395 w466 w472]
          tunnel: [w375 _ w466 w472] -> w361
          tunnel: [w376 w391 w465 w473] -> w359
          tunnel: w360 -> [w376 w392 w465 w473]
          tunnel: [_ w395 _ _] -> _
          tunnel: w358 -> [_ _ w449 _]
          tunnel: w357 -> [_ _ w446 _]
          tunnel: w356 -> [_ w389 w443 _]
          tunnel: w355 -> [_ _ w438 _]
          tunnel: w354 -> [_ w388 w433 _]
          tunnel: w353 -> [_ _ w416 _]
          tunnel: w352 -> [_ _ w415 _]
          tunnel: w351 -> [_ _ w414 _]
          tunnel: w350 -> [_ _ w413 _]
          tunnel: w349 -> [_ w387 _ _]
          tunnel: [_ w386 _ _] -> w348
          event "Intensity Graph": Cursor Move {
            n121 = event-data() -> ()  [unwired: 1 in, 7 out]
            n122 = property on="Intensity Graph" class="IntGraph (strict)"() -> ("Cursor.Cursor Y"=w383:dbl, "Cursor.Cursor X"=w379:dbl)  [unwired: 2 in, 2 out]
            n123 = Round Toward -Infinity(1:w383) -> (0:w380:dbl)
            n124 = Decrement(x=w380) -> (x-1=w382:dbl)
            n125 = local write "Run"(w380) -> ()
            n126 = Index Array(array=w381, index (row)=w382) -> (element=w384:ext[])  [unwired: 1 in]
            n127 = Bundle(w385, w384) -> (w377:cluster{ext[], ext[]})  [unwired: 1 in]
            n128 = Build Array(w377, w375) -> (w378:cluster{ext[], ext[]}[])
            n129 = local write "Histogram"(w378) -> ()
            n130 = property on="Histogram" class="XYGraph (strict)"("Cursor.Cursor X"=w379) -> ()  [unwired: 2 in, 2 out]
          }
          event "generator_enable": Value Change {
            n131 = event-data() -> ("NewVal"=w390:bool)  [unwired: 1 in, 5 out]
            n132 = call <instrlib>:"Configure RF.vi"("Power Level (-30.0)"=w388, "error in (no error)"=w387, "Frequency (1.0e9)"=w389, "VISA resource name"=w392) -> ("error out"=w394:errorcluster, "VISA resource name out"=w393:refnum<visa-resource-name>)  [unwired: 6 in]
            n133 = call <instrlib>:"Configure Output Enabled.vi"("error in (no error)"=w394, "Output Enabled (Off)"=w390, "VISA resource name"=w393) -> ("error out"=w386:errorcluster, "VISA resource name out"=w391:refnum<visa-resource-name>)  [unwired: 7 in]
          }
          event "Save": Value Change {
            n134 = event-data() -> ()  [unwired: 1 in, 6 out]
            n135 = Number To Fractional String(number=w449, precision (6)=i16 0) -> (F-format string=w450:string)  [unwired: 2 in]
            n136 = Number To Fractional String(number=w446, precision (6)=i16 0) -> (F-format string=w447:string)  [unwired: 2 in]
            n137 = Number To Fractional String(number=w443, precision (6)=i16 0) -> (F-format string=w444:string)  [unwired: 2 in]
            n138 = Number To Fractional String(number=w438, precision (6)=i16 3) -> (F-format string=w440:string)  [unwired: 2 in]
            n139 = Concatenate Strings("Step size [Hz] = ", w450, "\r\n") -> (w412:string)
            n140 = Concatenate Strings("Freq start [Hz] = ", w444, "\r\n") -> (w410:string)
            n141 = Concatenate Strings("Dwell time [s] = ", w440, "\r\n") -> (w409:string)
            n142 = Concatenate Strings("Freq stop [Hz] = ", w447, "\r\n") -> (w411:string)
            n143 = Concatenate Strings(w412, w411, w410, w409) -> (w405:string)
            n144 = Get Date/Time In Seconds() -> (seconds since 1Jan1904=w471:timestamp)
            n145 = Format Date/Time String(time format string (%c)="%Y-%m-%d_%H-%M-%S", seconds (now)=w471) -> (date/time string=w470:string)  [unwired: 1 in]
            n146 = Number To Fractional String(number=w433, precision (6)=i16 0) -> (F-format string=w435:string)  [unwired: 2 in]
            n147 = Number To Fractional String(number=w416, precision (6)=i16 3) -> (F-format string=w427:string)  [unwired: 2 in]
            n148 = Number To Fractional String(number=w415, precision (6)=i16 3) -> (F-format string=w424:string)  [unwired: 2 in]
            n149 = Number To Fractional String(number=w414, precision (6)=i16 3) -> (F-format string=w418:string)  [unwired: 2 in]
            n150 = Concatenate Strings(w470, ".dsp") -> (w398:string)
            "File name" <- w398
            n151 = Concatenate Strings("Power [dBm] = ", w435, "\r\n") -> (w404:string)
            n152 = Concatenate Strings("Position X [V] = ", w427, "\r\n") -> (w403:string)
            n153 = Concatenate Strings("Position Y [V] = ", w424, "\r\n") -> (w402:string)
            n154 = Concatenate Strings("Position Z [V] = ", w418, "\r\n") -> (w401:string)
            n155 = Concatenate Strings("D:\\Data\\raw data\\", w398) -> (w396:string)
            n156 = Array To Spreadsheet String(array=w461, 3:"%.0f" ("format string")) -> (spreadsheet string=w460:string)  [unwired: 1 in]
            n157 = Array To Spreadsheet String(array=w464, 3:"%.3f" ("format string")) -> (spreadsheet string=w458:string)  [unwired: 1 in]
            n158 = String To Path(string=w396) -> (path=w467:path)
            n159 = Number To Fractional String(number=w413, precision (6)=i16 0) -> (F-format string=w432:string)  [unwired: 2 in]
            n160 = Concatenate Strings(w460, "\r\n", w458) -> (w407:string)
            n161 = Concatenate Strings("Repetitions = ", w432, "\r\n") -> (w400:string)
            n162 = Concatenate Strings(w405, w404, w403, w402, w401, w400, "\r\n") -> (w406:string)
            n163 = Concatenate Strings(w406, w407) -> (w408:string)
            n164 = call <vilib>:"Write Characters To File.vi"("character string"=w408, "file path (dialog if empty)"=w467) -> ()  [unwired: 3 in, 1 out]
          }
          event Timeout {
            n165 = event-data() -> ()  [unwired: 1 in, 3 out]
          }
        }
        n166 = Not(x="start") -> (.not. x?=w372:bool)
        n167 = Select(t=w374, s=w372, f=T3."Set Variables") -> (s? t:f=w373:T3)
      }
    }
    n168 = Not(x="stop") -> (.not. x?=w50:bool)
    n169 = Select(t=w48, s=w50, f=T3."close") -> (s? t:f=w47:T3)
  }
